vi "set_sensor_auto-z.vi"(8 "error in (no error)":errorcluster, 9 "Auto-Z":bool, 10 "Sensor number":u8, 11 "VISA resource name":refnum<visa-resource-name>) -> (0 "error out":errorcluster, 3 "VISA resource name out":refnum<visa-resource-name>)   [LabVIEW 2018]
doc: "Automatically determine the Z-ratio of a sensor."
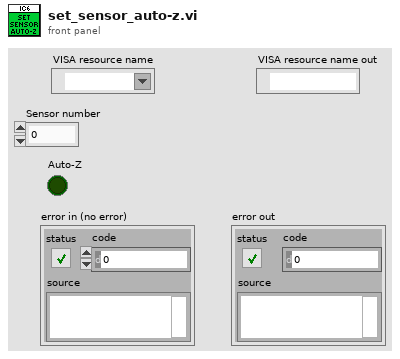
[diagram p1: front panel]
types:
  T1 = enum16{"Source", "General", "Input name", "Process name", "Logic", "Material", "Material name", "Output name", "Process", "Sensor", "Output type", "User message", "Layer", ""}
  T2 = enum16{"Hello", "Query", "Remote action", "Status", "Update"}
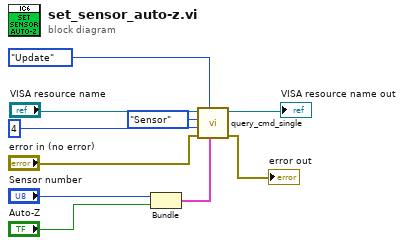
[diagram p0: block diagram]
diagram:
  n1 = Bundle("Sensor number"="Sensor number", "Auto-Z"="Auto-Z") -> (w4:cluster{"Sensor number":u8, "Auto-Z":bool})  [unwired: 1 in]
  n2 = call "query_cmd_single.vi"("Parameter"=w4, "Command group"=T2."Update", "error in (no error)"="error in (no error)", "Command ID"=u8 4, "Command subgroup"=T1."Sensor", "VISA resource name"="VISA resource name") -> ("error out"=→"error out":errorcluster, "VISA resource name out"=→"VISA resource name out":refnum<visa-resource-name>)  [unwired: 1 in, 3 out]
